vi "SeqnPanel_sm.vi"(10 "Seqn in":refnum<class "Sequence.lvclass">, 11 "Panel Refnum":refnum<vi>) -> ()   [LabVIEW 2012, in "StimulCtrls.lvlib"]
uses:
  StimulCtrls.lvlib
  Cohort.lvclass
  Sequence.lvclass
  UserControl/ElectdTerminal.ctl
  UserControl/Cohort_sm.ctl
panel:
  in  "Simplified Panel":T1
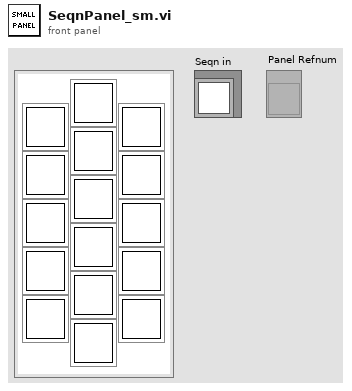
[diagram p1: front panel]
types:
  T1 = typedef "StimulCtrls.lvlib/Cohort_sm.ctl" = cluster{"T 5":T2, "T 6":T2, "T 7":T2, "T 8":T2, "T 9":T2, "T 10":T2, "T 11":T2, "T 12":T2, "T 13":T2, "T 14":T2, "T 15":T2, "T 0":T2, "T 1":T2, "T 2":T2, "T 3":T2, "T 4":T2}
  T2 = typedef "StimulCtrls.lvlib/ElectdTerminal.ctl" = u8
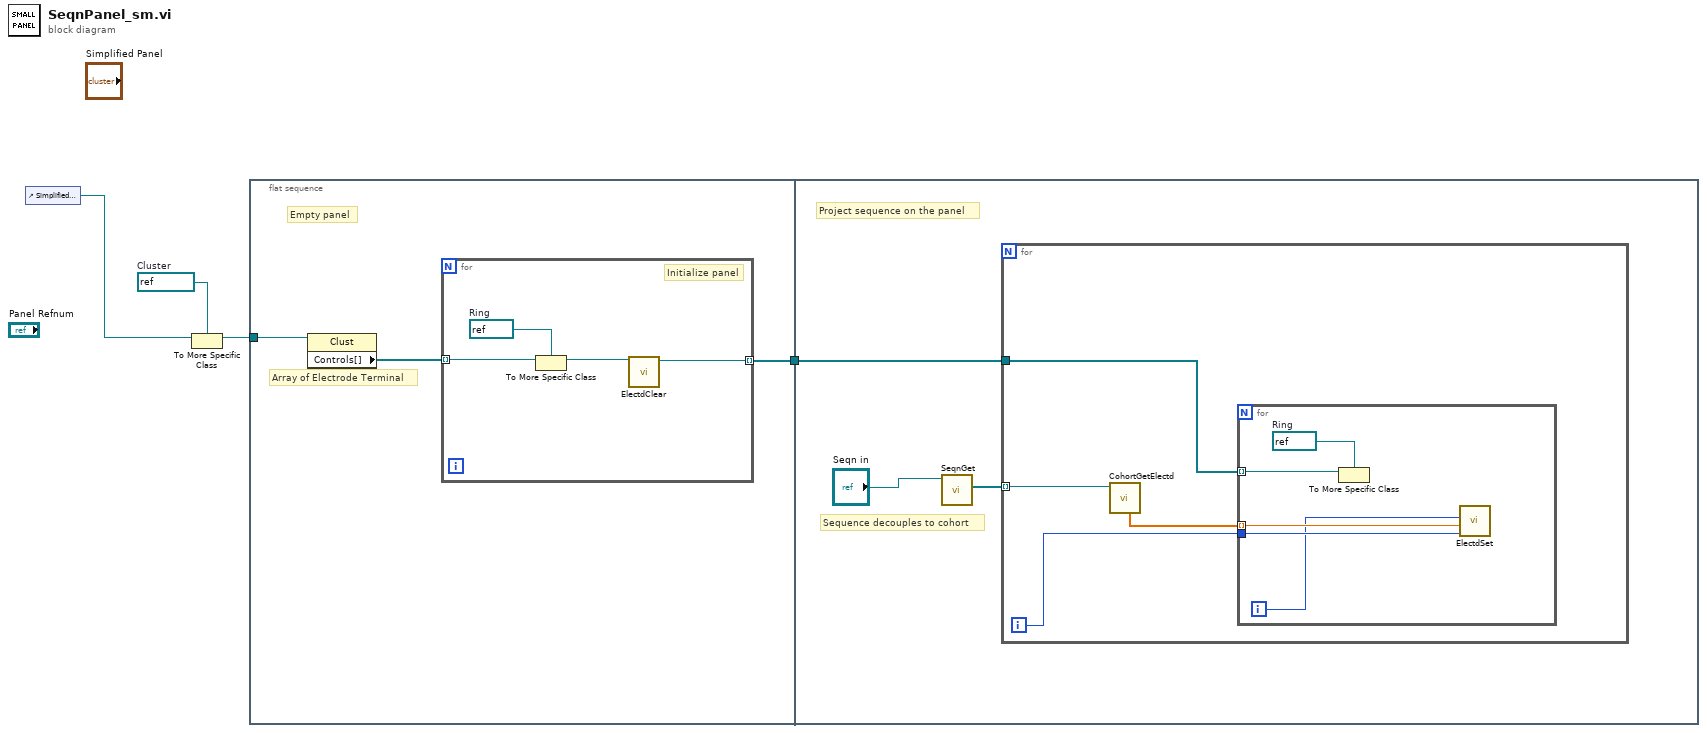
[diagram p0: block diagram]
diagram:
  w2 = refnum<vi> refnum  # Cluster
  n1 = control-ref of="Simplified Panel"() -> (w1:refnum<vi>)
  n2 = To More Specific Class(target class=w2, reference=w1) -> (specific class reference=w3:refnum<vi>)  [unwired: 1 in, 1 out]
  n3 = flat-sequence {
    tunnel: w3 -> [w7]
    tunnel: [w5] -> w4
    tunnel: w4 -> [w12]
    frame #0 {
      # "Empty panel"
      # "Array of Electrode Terminal"
      n4 = property class="Clust"(reference=w7) -> ("Controls[]"=w6:refnum<vi>[])  [unwired: 1 in, 2 out]
      n5 = for {
        tunnel: w6 -> [w11] mode=indexing
        tunnel: [w9] -> w5 mode=indexing
        w10 = refnum<vi> refnum  # Ring
        # "Initialize panel"
        n6 = To More Specific Class(target class=w10, reference=w11) -> (specific class reference=w8:refnum<vi>)  [unwired: 1 in, 1 out]
        n7 = call "ElectdClear.vi"("Electd in"=w8) -> ("Electd out"=w9:refnum<vi>)  [unwired: 10 in]
      }
    }
    frame #1 {
      # "Sequence decouples to cohort"
      # "Project sequence on the panel"
      n8 = call-dynamic "SeqnGet.vi"("Sequence in"="Seqn in") -> ("Cohorts"=w13:refnum<class "Cohort.lvclass">[])  [unwired: 8 in, 2 out]
      n9 = for {
        tunnel: w13 -> [w18] mode=indexing
        tunnel: w12 -> [w15]
        i -> [w16]
        n10 = call-dynamic "CohortGetElectd.vi"("Cohort in"=w18) -> ("Amplitude"=w17:sgl[])  [unwired: 6 in, 4 out]
        n11 = for {
          tunnel: w17 -> [w23] mode=indexing
          tunnel: w16 -> [w22]
          tunnel: w15 -> [w20] mode=indexing
          i -> [w21]
          w19 = refnum<vi> refnum  # Ring
          n12 = To More Specific Class(target class=w19, reference=w20) -> ()  [unwired: 1 in, 2 out]
          n13 = call "ElectdSet.vi"("Group #"=w22, "Amplitude"=w23, "Index"=w21) -> ()  [unwired: 8 in, 1 out]
        }
      }
    }
  }
